vi "Get_Image_PixelMap.vi"(11 "Image Data":T1) -> (3 "Image PixelMap":u32[][](array[numeric]))   [LabVIEW 2020]
uses:
  <vilib>/picture/picture.llb/imagedata.ctl
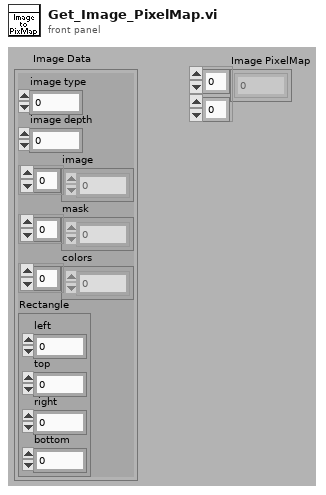
[diagram p1: front panel]
types:
  T1 = typedef "imagedata.ctl" = cluster{"image type":i32, "image depth":i32, "image":u8[], "mask":u8[], "colors":u32[], "Rectangle":cluster{"left":i16, "top":i16, "right":i16, "bottom":i16}}
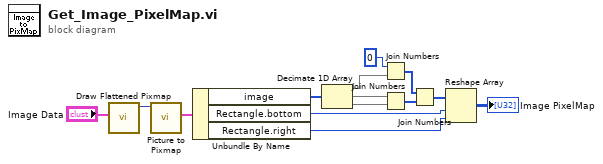
[diagram p0: block diagram]
diagram:
  n1 = call <vilib>:"Draw Flattened Pixmap.vi"("image data"="Image Data") -> ("new picture"=w14:picture)  [unwired: 8 in]
  n2 = call <vilib>:"Picture to Pixmap.vi"("picture"=w14) -> ("image data"=w12:T1)  [unwired: 9 in, 1 out]
  n3 = Unbundle By Name(w12) -> ("image"=w11:u8[], "Rectangle.bottom"=w10:i16, "Rectangle.right"=w9:i16)
  n4 = Decimate 1D Array(w11) -> (w6:u8[], w5:u8[], w4:u8[])
  n5 = Join Numbers(hi=u8 0 ("element"), lo=w6) -> ((hi.lo)=w3:u16[])
  n6 = Join Numbers(hi=w5, lo=w4) -> ((hi.lo)=w2:u16[])
  n7 = Join Numbers(hi=w3, lo=w2) -> ((hi.lo)=w1:u32[])
  n8 = Reshape Array(w1, w10, w9) -> (→"Image PixelMap":u32[][])
